vi "Tbl_Remove (SubVI).vi"(11 "Table in":refnum<vi>) -> (3 "element":i32)   [LabVIEW 2017]
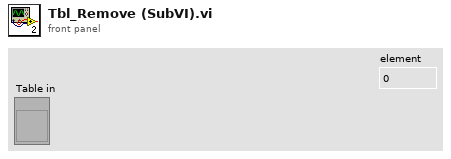
[diagram p1: front panel]
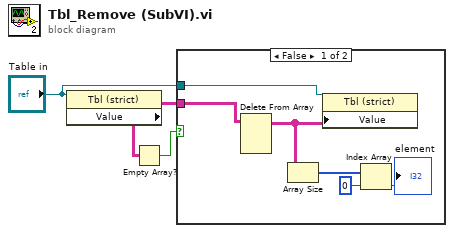
[diagram p0: block diagram]
diagram:
  n1 = property class="Tbl (strict)"(reference="Table in") -> ("Value"=w3:string[][])  [unwired: 1 in, 2 out]
  n2 = Empty Array?(array=w3) -> (empty?=w2:bool)
  n3 = case shown="False" w2 {
    tunnel: w3 -> [w9 _]
    tunnel: "Table in" -> [w8 _]
    frame False {
      n4 = Delete From Array(array=w9) -> (array with subset deleted=w7:string[][])  [unwired: 3 in, 1 out]
      n5 = Array Size(array=w7) -> (size(s)=w6:i32[])
      n6 = property class="Tbl (strict)"(reference=w8, "Value"=w7) -> ()  [unwired: 1 in, 2 out]
      n7 = Index Array(array=w6, index=0) -> (element=→"element":i32)
    }
    frame True {
    }
  }
